vi "NT Write Boolean_On Change.vi"(8 "error in":errorcluster, 9 "Boolean":bool, 11 "Name":string="Boolean") -> (0 "error out":errorcluster)   [LabVIEW 2020]
uses:
  <vilib>/Rock Robotics/Network Tables/NT Write Boolean.vi
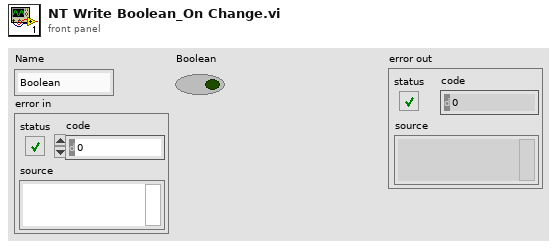
[diagram p1: front panel]
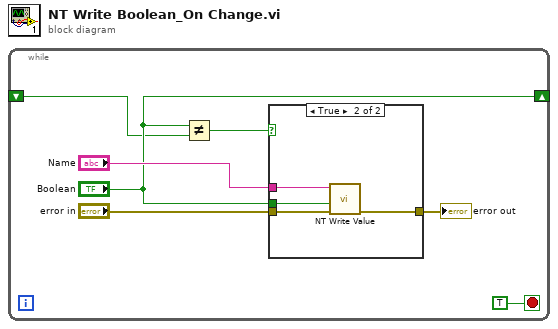
[diagram p0: block diagram]
diagram:
  n1 = while {
    shift-right: ["Boolean"] -> _
    shift-left: _ -> [w3]
    stop <- TRUE stop-if-true
    n2 = Not Equal?(x="Boolean", y=w3) -> (x != y?=w2:bool)
    n3 = case shown="True" w2 {
      tunnel: "Name" -> [_ w12]
      tunnel: "error in" -> [w8 w11]
      tunnel: [w8 w10] -> w5
      tunnel: "Boolean" -> [_ w9]
      frame False {
      }
      frame True {
        n4 = call-poly <vilib>:"NT Write Value.vi"("error in"=w11, "Boolean"=w9, "Name"=w12) -> ("error out"=w10:errorcluster)  [unwired: 8 in]
      }
    }
    "error out" <- w5
  }
